vi "CreateSignal.vi"(0 "Signal in":refnum<class "Signal.lvclass">, 5 "error in (no error)":errorcluster, 12 "Tags":T1, 13 "Logger":refnum<class "Logger.lvclass">) -> (14 "Signal out":refnum<class "Signal.lvclass">, 19 "error out":errorcluster)   [LabVIEW 2019, in "Signal.lvclass"]
uses:
  Signal.lvclass
  D:/GIT H4000/H4000/src/Proccess_class/Proccess.lvclass
  Proccess_class/TAGs.ctl
  Logger_class/Logger.lvclass
  Proccess_class/Proccess.lvclass
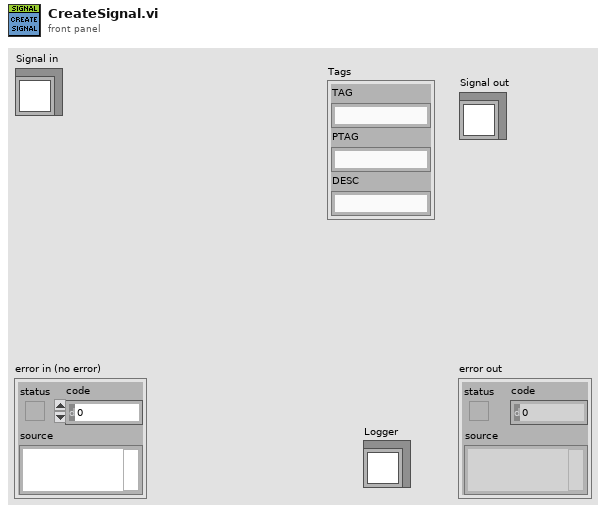
[diagram p1: front panel]
types:
  T1 = typedef "Proccess.lvclass/TAGs.ctl" = cluster{"TAG":string, "PTAG":string, "DESC":string}
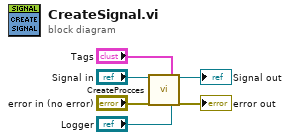
[diagram p0: block diagram]
diagram:
  n1 = call "CreateProcces.vi"("reference in"="Signal in", "error in (no error)"="error in (no error)", "Tags"="Tags", "Logger"="Logger") -> ("reference out"=→"Signal out":refnum<class "Signal.lvclass">, "error out"=→"error out":errorcluster)  [unwired: 14 in]
